vi "Get File Path.vi"(11 "FileName":string="Config") -> (3 "FilePath":path)   [LabVIEW 2015]
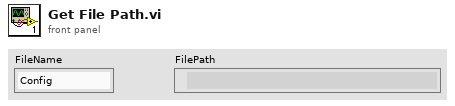
[diagram p1: front panel]
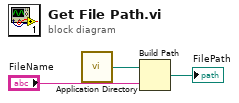
[diagram p0: block diagram]
diagram:
  n1 = call <vilib>:"Application Directory.vi"() -> ("Application Directory"=w1:path)
  n2 = Build Path(base path=w1, name or relative path="FileName") -> (appended path=→"FilePath":path)
